vi "AudioTest.Waveform to Plot Item.vi"(8 "error in":errorcluster, 10 "Plot Template":T1, 11 "Waveform":waveform(dbl)) -> (0 "error out":errorcluster, 2 "Plot Item":T1)   [LabVIEW 2018]
uses:
  TypeDefs/AudioTest.Result Plot Data.ctl
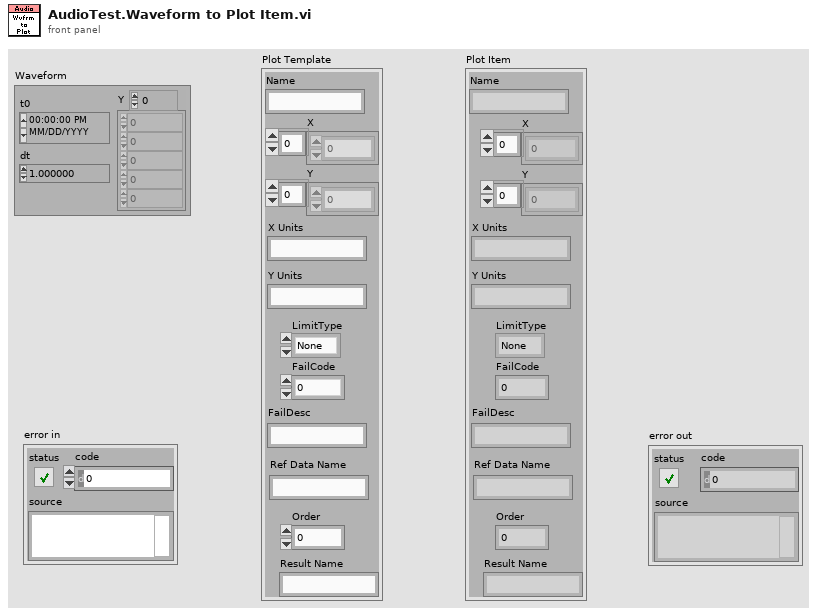
[diagram p1: front panel]
types:
  T1 = typedef "AudioTest.Result Plot Data.ctl" = cluster{"Order":i32, "Name":string, "X":dbl[], "Y":dbl[], "X Units":string, "Y Units":string, "LimitType":enum16{"None", "LL", "UL"}, "FailCode":i32, "FailDesc":string, "Ref Data Name":string, "Result Name":string}
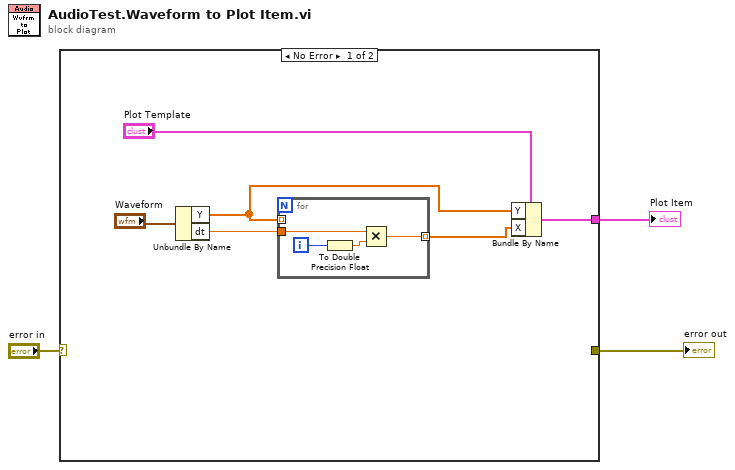
[diagram p0: block diagram]
diagram:
  n1 = case shown="No Error" "error in" {
    selector: "error in" -> [_ w14]
    tunnel: [_ w14] -> w2
    tunnel: [w5 _] -> w1
    frame No Error {
      n2 = Unbundle By Name("Waveform") -> ("Y"=w4:dbl[], "dt"=w8:dbl)
      n3 = for {
        tunnel: w8 -> [w13]
        tunnel: [w10] -> w6 mode=indexing
        tunnel: w4 -> [_] mode=indexing
        i -> [w11]
        n4 = To Double Precision Float(number=w11) -> (double precision float=w12:dbl)
        n5 = Multiply(x=w13, y=w12) -> (x*y=w10:dbl)
      }
      n6 = Bundle By Name(cluster="Plot Template", "Y"=w4, "X"=w6) -> (w5:T1)
    }
    frame Error {
    }
  }
  "error out" <- w2
  "Plot Item" <- w1
